vi "32datapack.vi"(11 "脉冲信息":T1(array[cluster])=[[{"幅值"=2.0, "频率"=31, "脉宽"=20, "选通"=FALSE, "脉宽单位"=enum."ms", "字符串"="CH0", "时间"=0}, {"幅值"=2.0, "频率"=31, "脉宽"=20, "选通"=FALSE, "脉宽单位"=enum."us", "字符串"="CH1", "时间"=0}, {"幅值"=1.0, "频率"=31, "脉宽"=90, "选通"=FALSE, "脉宽单位"=enum."ns", "字符串"="CH2", "时间"=0}, {"幅值"=1.0, "频率"=31, "脉宽"=20, "选通"=TRUE, "脉宽单位"=enum."us", "字符串"="CH3", "时间"=0}, {"幅值"=2.0, "频率"=31, "脉宽"=20, "选通"=FALSE, "脉宽单位"=enum."us", "字符串"="CH4", "时间"=0}, {"幅值"=3.0, "频率"=31, "脉宽"=20, "选通"=FALSE, "脉宽单位"=enum."us", "字符串"="CH5", "时间"=0}, {"幅值"=2.0, "频率"=31, "脉宽"=20, "选通"=FALSE, "脉宽单位"=enum."us", "字符串"="CH6", "时间"=0}, {"幅值"=10.0, "频率"=31, "脉宽"=20, "选通"=FALSE, "脉宽单位"=enum."us", "字符串"="CH7", "时间"=0}], [{"幅值"=1.0, "频率"=31, "脉宽"=20, "选通"=FALSE, "脉宽单位"=enum."us", "字符串"="CH8", "时间"=0}, {"幅值"=1.0, "频率"=31, "脉宽"=20, "选通"=FALSE, "脉宽单位"=enum."us", "字符串"="CH9", "时间"=0}, {"幅值"=1.0, "频率"=31, "脉宽"=20, "选通"=FALSE, "脉宽单位"=enum."us", "字符串"="CH10", "时间"=0}, {"幅值"=1.0, "频率"=31, "脉宽"=20, "选通"=FALSE, "脉宽单位"=enum."us", "字符串"="CH11", "时间"=0}, {"幅值"=1.0, "频率"=31, "脉宽"=20, "选通"=TRUE, "脉宽单位"=enum."us", "字符串"="CH12", "时间"=0}, {"幅值"=1.0, "频率"=31, "脉宽"=20, "选通"=FALSE, "脉宽单位"=enum."us", "字符串"="CH13", "时间"=0}, {"幅值"=1.0, "频率"=31, "脉宽"=20, "选通"=FALSE, "脉宽单位"=enum."us", "字符串"="CH14", "时间"=0}, {"幅值"=1.0, "频率"=31, "脉宽"=20, "选通"=FALSE, "脉宽单位"=enum."us", "字符串"="CH15", "时间"=0}], [{"幅值"=1.0, "频率"=31, "脉宽"=20, "选通"=FALSE, "脉宽单位"=enum."us", "字符串"="CH16", "时间"=0}, {"幅值"=1.0, "频率"=31, "脉宽"=20, "选通"=FALSE, "脉宽单位"=enum."us", "字符串"="CH17", "时间"=0}, {"幅值"=1.0, "频率"=31, "脉宽"=20, "选通"=FALSE, "脉宽单位"=enum."us", "字符串"="CH18", "时间"=0}, {"幅值"=1.0, "频率"=31, "脉宽"=20, "选通"=TRUE, "脉宽单位"=enum."us", "字符串"="CH19", "时间"=0}, {"幅值"=1.0, "频率"=31, "脉宽"=20, "选通"=FALSE, "脉宽单位"=enum."us", "字符串"="CH20", "时间"=0}, {"幅值"=1.0, "频率"=31, "脉宽"=20, "选通"=TRUE, "脉宽单位"=enum."us", "字符串"="CH21", "时间"=0}, {"幅值"=1.0, "频率"=31, "脉宽"=20, "选通"=FALSE, "脉宽单位"=enum."us", "字符串"="CH22", "时间"=0}, {"幅值"=1.0, "频率"=31, "脉宽"=20, "选通"=FALSE, "脉宽单位"=enum."us", "字符串"="CH23", "时间"=0}], [{"幅值"=1.0, "频率"=31, "脉宽"=20, "选通"=TRUE, "脉宽单位"=enum."us", "字符串"="CH24", "时间"=0}, {"幅值"=1.0, "频率"=31, "脉宽"=20, "选通"=FALSE, "脉宽单位"=enum."us", "字符串"="CH25", "时间"=0}, {"幅值"=1.0, "频率"=31, "脉宽"=20, "选通"=TRUE, "脉宽单位"=enum."us", "字符串"="CH26", "时间"=0}, {"幅值"=1.0, "频率"=31, "脉宽"=20, "选通"=FALSE, "脉宽单位"=enum."us", "字符串"="CH27", "时间"=0}, {"幅值"=1.0, "频率"=31, "脉宽"=20, "选通"=FALSE, "脉宽单位"=enum."us", "字符串"="CH28", "时间"=0}, {"幅值"=1.0, "频率"=31, "脉宽"=20, "选通"=FALSE, "脉宽单位"=enum."us", "字符串"="CH29", "时间"=0}, {"幅值"=1.0, "频率"=31, "脉宽"=20, "选通"=FALSE, "脉宽单位"=enum."us", "字符串"="CH30", "时间"=0}, {"幅值"=1.0, "频率"=31, "脉宽"=20, "选通"=TRUE, "脉宽单位"=enum."us", "字符串"="CH31", "时间"=0}]] {"脉宽" min=1 step=1; "幅值" min=0 max=15 step=0.1 format="%#_3f"}) -> (3 "字符串":string)   [LabVIEW 2018]
panel:
  # "V"
  # "Hz"
  # "s"
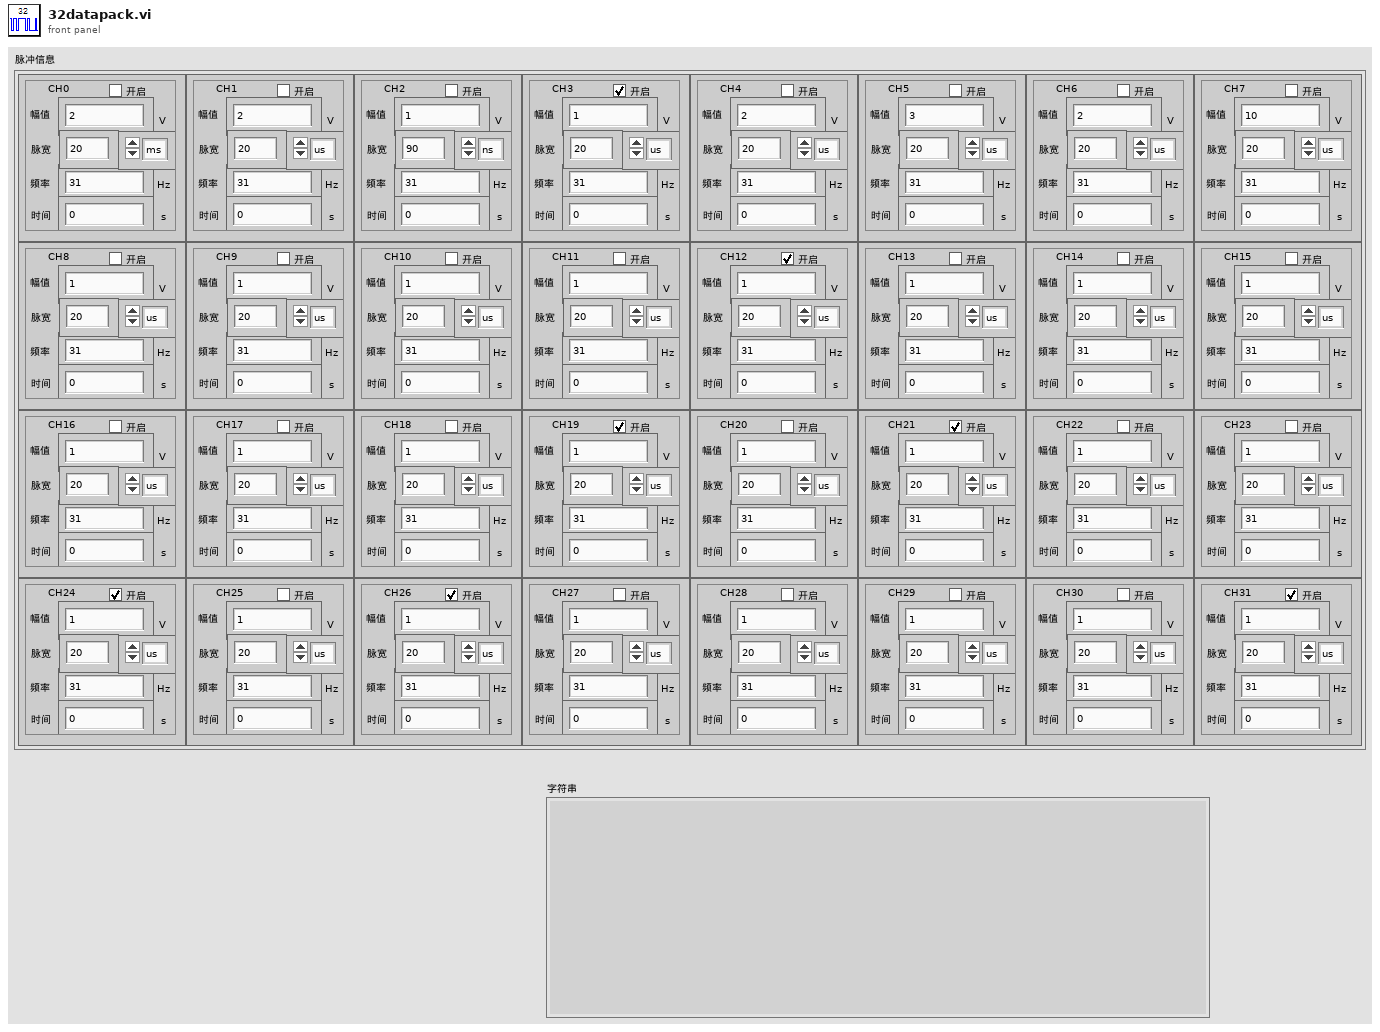
[diagram p1: front panel]
types:
  T1 = cluster{"幅值":sgl, "频率":u32, "脉宽":u16, "选通":bool, "脉宽单位":enum16{"ns", "us", "ms"}, "字符串":string, "时间":i32}[][]
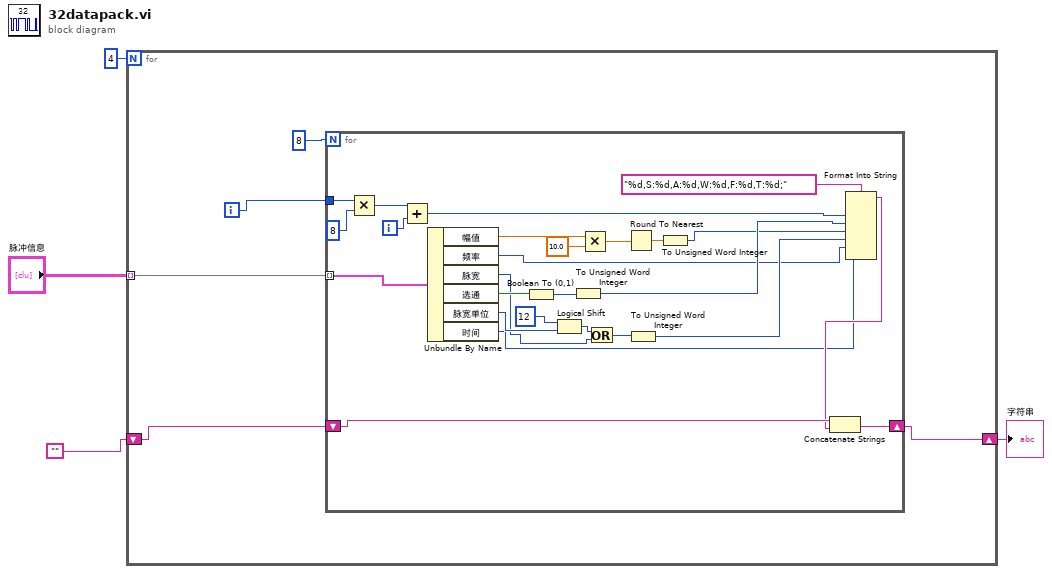
[diagram p0: block diagram]
diagram:
  n1 = for {
    N: 4 -> [_]
    tunnel: "脉冲信息" -> [w8] mode=indexing
    shift-right: [w6] -> w1
    shift-left: "" -> [w7]
    i -> [w5]
    n2 = for {
      N: 8 -> [_]
      tunnel: w8 -> [w35] mode=indexing
      shift-right: [w28] -> w6
      shift-left: w7 -> [w27]
      tunnel: w5 -> [w33]
      i -> [w31]
      n3 = Multiply(x=w33, y=8) -> (x*y=w30:i32)
      n4 = Add(x=w30, y=w31) -> (x+y=w29:i32)
      n5 = Unbundle By Name(w35) -> ("幅值"=w22:sgl, "频率"=w11:u32, "脉宽"=w14:u16, "选通"=w25:bool, "脉宽单位"=w17:enum16{"ns", "us", "ms"}, "时间"=w10:i32)
      n6 = Boolean To (0,1)(Boolean=w25) -> (0, 1=w24:i16)
      n7 = Logical Shift(y=i16 12, x=w17) -> (x << y=w15:u32)
      n8 = To Unsigned Word Integer(number=w24) -> (unsigned 16bit integer=w23:u16)
      n9 = Multiply(x=w22, y=sgl 10.0) -> (x*y=w20:sgl)
      n10 = Or(x=w15, y=w14) -> (x .or. y?=w13:u32)
      n11 = Round To Nearest(number=w20) -> (nearest integer value=w19:sgl)
      n12 = To Unsigned Word Integer(number=w13) -> (unsigned 16bit integer=w12:u16)
      n13 = To Unsigned Word Integer(number=w19) -> (unsigned 16bit integer=w18:u16)
      n14 = Format Into String(format string="%d,S:%d,A:%d,W:%d,F:%d,T:%d;" ("格式字符串"), w29, w23, w18, w12, w11, w10) -> (resulting string=w26:string)  [unwired: 2 in, 1 out]
      n15 = Concatenate Strings(w27, w26) -> (w28:string)
    }
  }
  "字符串" <- w1
